vi "Save_Displacement_in_Array(Track)-1.vi"(2 "[IN] Index for Collect":i32, 3 "[IN] Collecting Array":dbl[](array[numeric]), 4 "[IN] Index of displ":i32, 5 "[IN]Source Array":dbl[](array[numeric])) -> (0 "[OUT] Finish Index for Collect":i32, 1 "[OUT] Collecting Array":dbl[](array[numeric]))   [LabVIEW 2013]
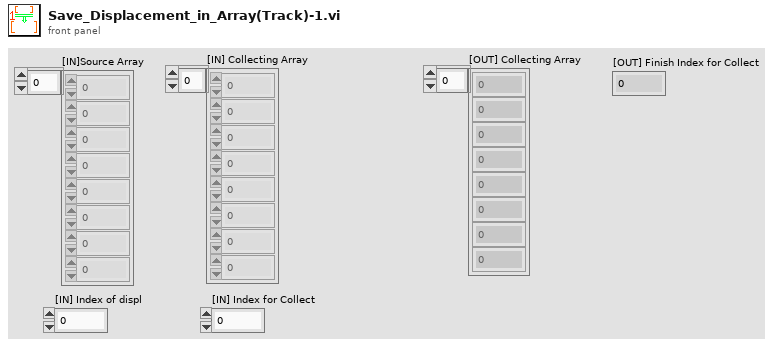
[diagram p1: front panel]
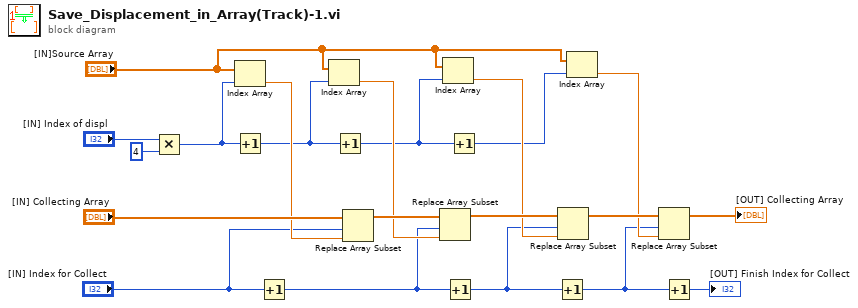
[diagram p0: block diagram]
diagram:
  n1 = Multiply(x="[IN] Index of displ", y=4) -> (x*y=w1:i32)
  n2 = Index Array(array="[IN]Source Array", index=w1) -> (element=w20:dbl)
  n3 = Increment(x=w1) -> (x+1=w16:i32)
  n4 = Increment(x="[IN] Index for Collect") -> (x+1=w14:i32)
  n5 = Index Array(array="[IN]Source Array", index=w16) -> (element=w17:dbl)
  n6 = Increment(x=w16) -> (x+1=w10:i32)
  n7 = Replace Array Subset(array="[IN] Collecting Array", new element=w20, index="[IN] Index for Collect") -> (w18:dbl[])
  n8 = Replace Array Subset(array=w18, new element=w17, index=w14) -> (w15:dbl[])
  n9 = Index Array(array="[IN]Source Array", index=w10) -> (element=w13:dbl)
  n10 = Increment(x=w14) -> (x+1=w11:i32)
  n11 = Increment(x=w10) -> (x+1=w9:i32)
  n12 = Increment(x=w11) -> (x+1=w6:i32)
  n13 = Replace Array Subset(array=w15, new element=w13, index=w11) -> (w12:dbl[])
  n14 = Index Array(array="[IN]Source Array", index=w9) -> (element=w7:dbl)
  n15 = Replace Array Subset(array=w12, new element=w7, index=w6) -> (→"[OUT] Collecting Array":dbl[])
  n16 = Increment(x=w6) -> (x+1=→"[OUT] Finish Index for Collect":i32)
